vi "PicoScope4000IsReady.vi"(8 "error in (no error)":errorcluster, 11 "handle in":i16) -> (0 "error out":errorcluster, 3 "handle out":i16, 6 "ready":i16)   [LabVIEW 2009]
doc: "Calls sIsReady"
uses:
  ps4000.dll
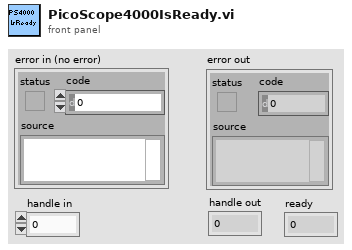
[diagram p1: front panel]
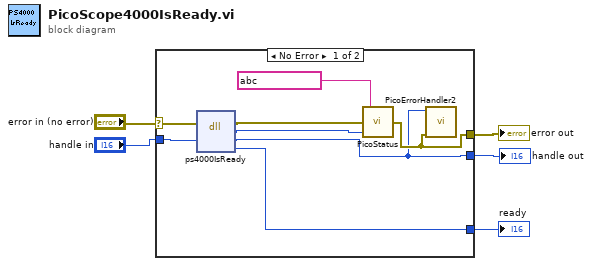
[diagram p0: block diagram]
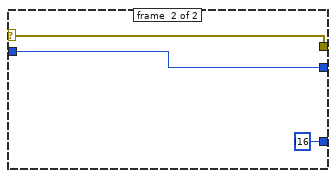
[diagram p2: hidden frame]
diagram:
  n1 = case shown="No Error" "error in (no error)" {
    selector: "error in (no error)" -> [w11 w15]
    tunnel: "handle in" -> [w10 w16]
    tunnel: [w7 w16] -> w5
    tunnel: [w12 w15] -> w4
    tunnel: [w6 i16 ? ("ready")] -> w3
    frame #0 {
      n2 = dll-call lib="PS4000.dll" fn="ps4000IsReady" ("ps3000.dll:_ps3000_open_unit@0")(error in=w11, "handle"=w10) -> (error out=w9:errorcluster, "PICO_STATUS"=w8:u32, "handle"=w7:i16, "ready"=w6:i16)  [unwired: 3 in, 1 out]
      n3 = call "PicoStatus.vi"("PICO STATUS"=w8, "error in"=w9, "source"=string ?) -> ("error out"=w12:errorcluster)
      n4 = call "PicoErrorHandler2.vi"("error in (no error)"=w12, "handle In"=w7) -> ()  [unwired: 9 in, 1 out]
    }
    frame #1 {
    }
  }
  "error out" <- w4
  "handle out" <- w5
  "ready" <- w3
